vi "Measurement Logic.vi"() -> ()   [LabVIEW 2021, in "channelGanging.lvlib"]
uses:
  channelGanging.lvlib
  Measurement Results.ctl
  Measurement Configuration.ctl
  <vilib>/MeasurementLink/MeasurementLink Measurement Server/Measure Call Context/Measure Call Context.lvclass
panel:
  out "measure call context out":refnum<class "Measure Call Context.lvclass">
  in  "measure call context in":refnum<class "Measure Call Context.lvclass">
  out "measurement results":T1
  in  "measurement configuration":T2={"Source channel names"=[], "Source resource names"=[], "Source channel mode"=[], "Source system configuration"=enum."Parallel", "Source voltage level"=2.0, "Source voltage level range"=20.0, "Source sense"=enum."Remote", "Source limit symmetry"=enum."Asymmetric", "Source current limit range"=2.0, "Source current limit low"=2.0, "Source current limit high"=20.0, "Source aperture time"=0.01, "Source transient response"=enum."Slow", "Load channel names"=[], "Load resource names"=[], "Load channel mode"=[], "Load system configuration"=enum."Parallel", "Load current Level"=2.0, "Load current level range"=20.0, "Load Sense"=enum."Remote", "Load limit symmetry"=enum."Asymmetric", "Load voltage limit range"=2.0, "Load voltage limit low"=2.0, "Load voltage limit high"=20.0, "Load aperture time"=0.01, "Load transient response"=enum."Slow", "Measurement time"=0.01} {"Measurement time" format="%.3p"; "Load aperture time" format="%.3p"; "Load voltage limit high" format="%#_6p"; "Load voltage limit low" format="%#_6p"; "Load voltage limit range" format="%#_6p"; "Load current level range" format="%#_6p"; "Load current Level" format="%#_6p"; "Source aperture time" format="%.3p"; "Source current limit high" format="%#_6p"; "Source current limit low" format="%#_6pA"; "Source current limit range" format="%#_6p"; "Source voltage level range" format="%#_6pV"; "Source voltage level" format="%#_6p"}
  out "error out":errorcluster
  in  "error in":errorcluster
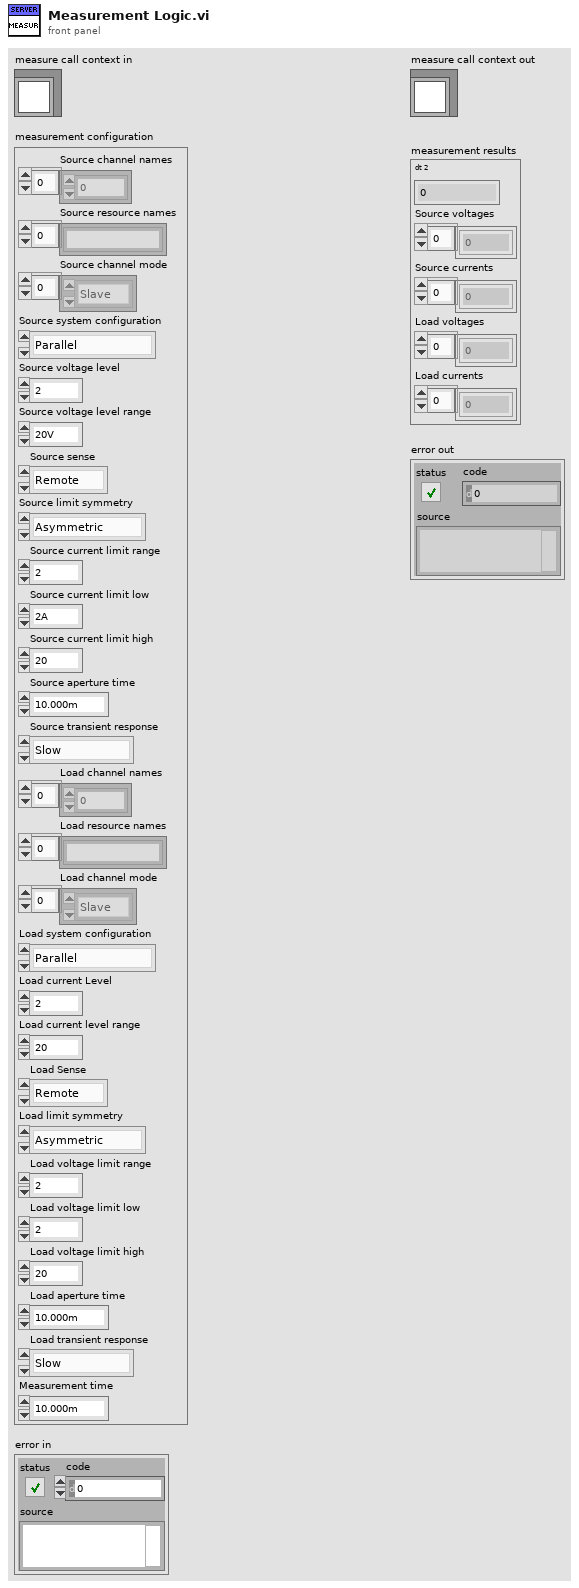
[diagram p1: front panel]
types:
  T1 = typedef "channelGanging.lvlib/Measurement Results.ctl" = cluster{"dt 2":dbl, "Source voltages":dbl[], "Source currents":dbl[], "Load voltages":dbl[], "Load currents":dbl[]}
  T2 = typedef "channelGanging.lvlib/Measurement Configuration.ctl" = cluster{"Source channel names":i32[], "Source resource names":string[], "Source channel mode":enum32{"Master", "Slave", "Slave- inverted"}[], "Source system configuration":enum32{"Parallel", "Series"}, "Source voltage level":dbl, "Source voltage level range":dbl, "Source sense":enum32{"Remote", "Local"}, "Source limit symmetry":enum32{"Asymmetric", "Symmetric"}, "Source current limit range":dbl, "Source current limit low":dbl, "Source current limit high":dbl, "Source aperture time":dbl, "Source transient response":enum32{"Fast", "Normal", "Slow"}, "Load channel names":i32[], "Load resource names":string[], "Load channel mode":enum32{"Master", "Slave", "Slave- inverted"}[], "Load system configuration":enum32{"Parallel", "Series"}, "Load current Level":dbl, "Load current level range":dbl, "Load Sense":enum32{"Remote", "Local"}, "Load limit symmetry":enum32{"Asymmetric", "Symmetric"}, "Load voltage limit range":dbl, "Load voltage limit low":dbl, "Load voltage limit high":dbl, "Load aperture time":dbl, "Load transient response":enum32{"Fast", "Normal", "Slow"}, "Measurement time":dbl}
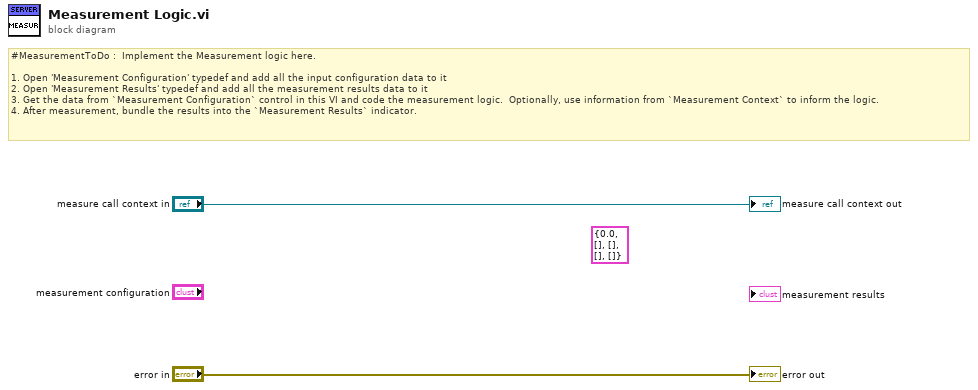
[diagram p0: block diagram]
diagram:
  (unwired) T1 {"dt 2"=0.0, "Source voltages"=[], "Source currents"=[], "Load voltages"=[], "Load currents"=[]} ("Measurement Results")
  # "#MeasurementToDo :  Implement the Measurement logic here.\n\n1. Open 'Measurement Configuration' typedef and add all the input configuration data to it\n2. Open 'Measurement Results' typedef and add all the measurement results data to it\n3. Get the data from `Measurement Configuration` control in this VI and code the measurement logic.  Optionally, use information from `Measurement Context` to inform the logic.\n4. After measurement, bundle the results into the `Measurement Results` indicator."
  "error out" <- "error in"
  "measure call context out" <- "measure call context in"
